vi "Set Base Path.vi"(8 "error in (no error)":errorcluster, 10 "Base Path":path, 11 "Log File Specification in":refnum<class "Log File Specification.lvclass">) -> (0 "error out":errorcluster, 3 "Log File Specification out":refnum<class "Log File Specification.lvclass">)   [LabVIEW 2015, in "Waveform Data Logger Shared.lvlib" / "Log File Specification.lvclass"]
doc: "Sets the base path for the log file, which is used to construct instance file paths based on the specified path tag values when the instance file is opened."
uses:
  Log File Specification.lvclass
  Log File Specification.lvclass/Log File Specification.ctl
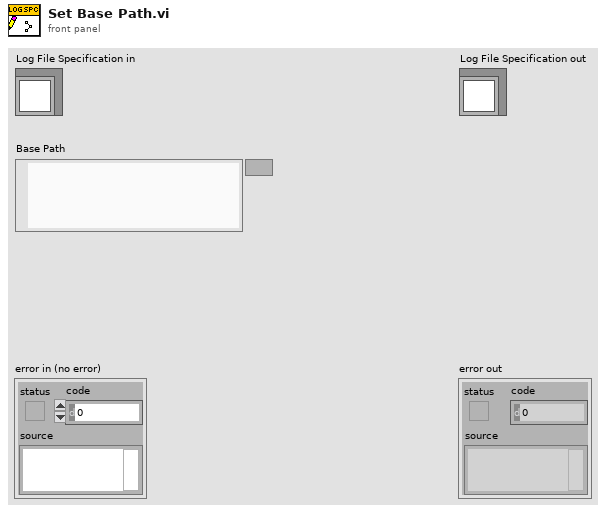
[diagram p1: front panel]
types:
  T1 = typedef "Waveform Data Logger Shared.lvlib/Log File Specification.lvclass/Path Segment.ctl" = cluster{"String":string, "Is Tag":bool}
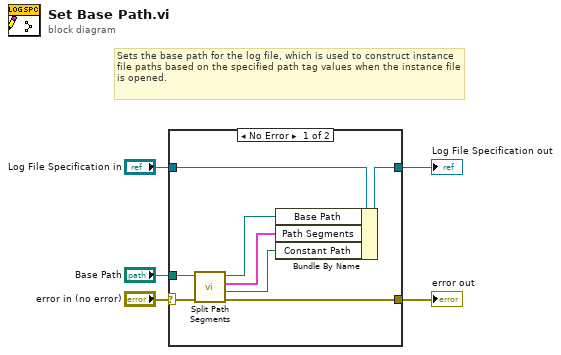
[diagram p0: block diagram]
diagram:
  # "Sets the base path for the log file, which is used to construct instance file paths based on the specified path tag values when the instance file is opened."
  n1 = case shown="No Error" "error in (no error)" {
    selector: "error in (no error)" -> [w13 w14]
    tunnel: "Log File Specification in" -> [w11 w15]
    tunnel: [w10 w15] -> w4
    tunnel: [w12 w14] -> w2
    tunnel: "Base Path" -> [w9 _]
    frame No Error {
      n2 = call "Split Path Segments.vi"("error in (no error)"=w13, "Base Path in"=w9) -> ("error out"=w12:errorcluster, "Constant Path"=w6:bool, "Path Segments"=w8:T1[], "Base Path out"=w7:path)  [unwired: 6 in]
      n3 = Bundle By Name(cluster=w11, "Base Path"=w7, "Path Segments"=w8, "Constant Path"=w6) -> (w10:refnum<class "Log File Specification.lvclass">)
    }
    frame Error {
    }
  }
  "error out" <- w2
  "Log File Specification out" <- w4
